vi "Flattened String to Variant.vi"(5 "variant in":refnum<class "variant.lvclass">, 8 "error in (no error)":errorcluster, 10 "data":refnum<class "DataString.lvclass">, 11 "type":refnum<class "TD.lvclass">) -> (0 "error out":errorcluster, 3 "variant out":refnum<class "variant.lvclass">)   [LabVIEW 2020, in "variant.lvlib" / "variant.lvclass"]
uses:
  variant.lvclass
  Type Descriptor/TD.lvclass
  DataString/DataString.lvclass
  variant.lvclass/variant.ctl
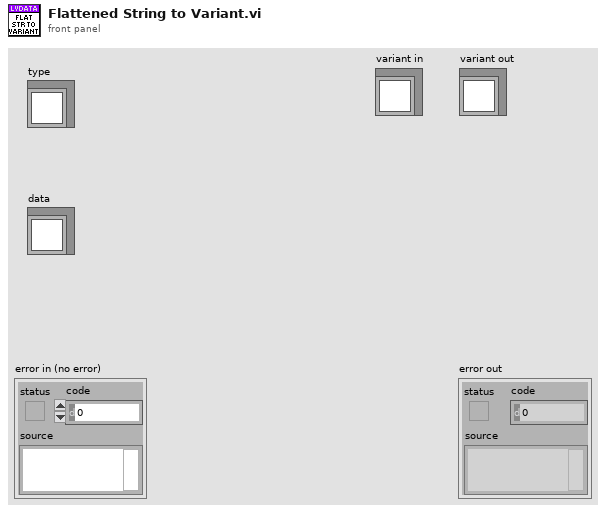
[diagram p1: front panel]
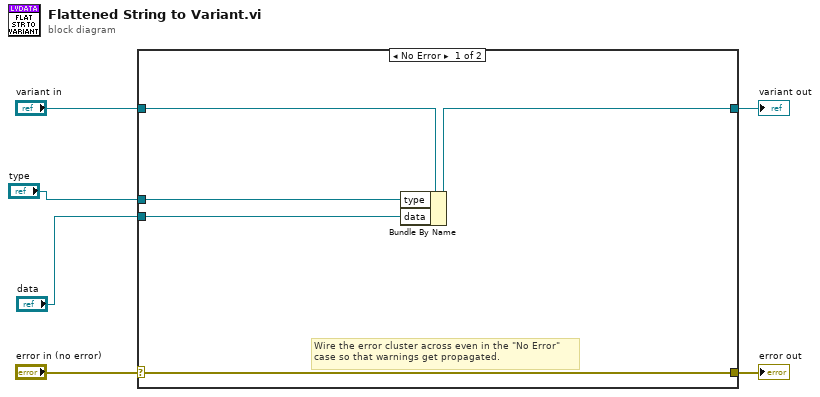
[diagram p0: block diagram]
diagram:
  n1 = case shown="No Error" "error in (no error)" {
    selector: "error in (no error)" -> [w11 w13]
    tunnel: [w11 w13] -> w5
    tunnel: [w10 w12] -> w3
    tunnel: "variant in" -> [w9 w12]
    tunnel: "data" -> [w8 _]
    tunnel: "type" -> [w7 _]
    frame No Error {
      # "Wire the error cluster across even in the \"No Error\"\ncase so that warnings get propagated."
      n2 = Bundle By Name(cluster=w9, "type"=w7, "data"=w8) -> (w10:refnum<class "variant.lvclass">)
    }
    frame Error {
    }
  }
  "error out" <- w5
  "variant out" <- w3
